vi "Find Resource by Type (U32).vi"(6 "Error if not found? (F)":bool, 8 "error in (no error)":errorcluster, 10 "Resource Type":u32, 11 "Resources":T2) -> (0 "error out":errorcluster, 1 "Index":i32, 2 "Found?":bool, 3 "Resource":T1)   [LabVIEW 2023]
uses:
  CTLs/Resource Array.ctl
  CTLs/Resource.ctl
  <vilib>/Utility/error.llb/Error Cluster From Error Code.vi
  <vilib>/ErrorRing/Error Ring.xnode
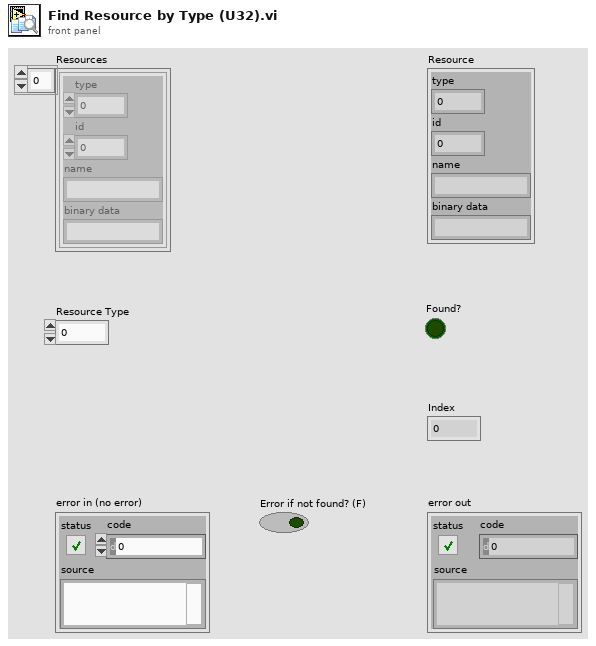
[diagram p1: front panel]
types:
  T1 = typedef "Resource.ctl" = cluster{"type":u32, "id":i32, "name":string, "binary data":string}
  T2 = typedef "Resource Array.ctl" = T1[]
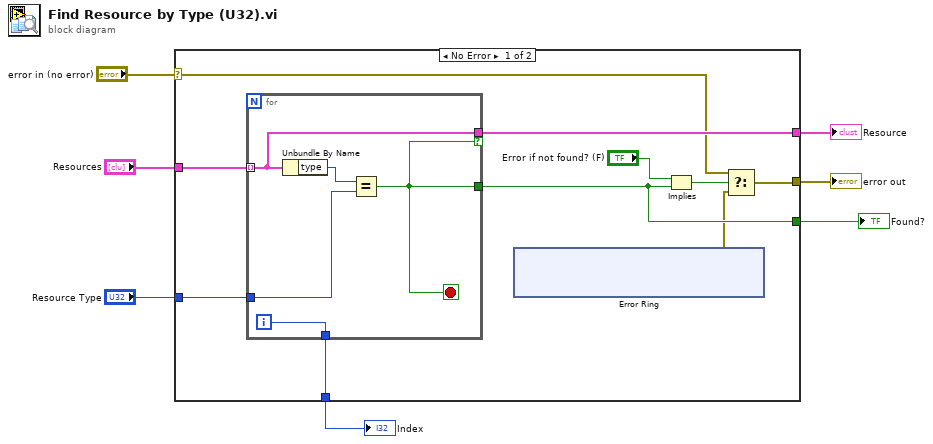
[diagram p0: block diagram]
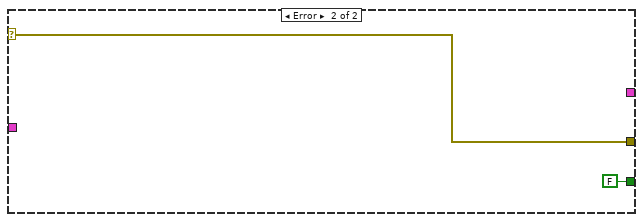
[diagram p2: hidden frame]
diagram:
  n1 = case shown="No Error" "error in (no error)" {
    selector: "error in (no error)" -> [w11 w28]
    tunnel: "Resources" -> [w17 _]
    tunnel: "Resource Type" -> [w16 _]
    tunnel: [w13 _] -> w5
    tunnel: [w12 _] -> w4
    tunnel: [w10 FALSE] -> w2
    tunnel: [w8 w28] -> w1
    frame No Error {
      n2 = for {
        tunnel: w17 -> [w24] mode=indexing
        tunnel: w16 -> [w25]
        tunnel: [w23] -> w10
        tunnel: [w24] -> w12 if=w23
        tunnel: [w22] -> w13
        i -> [w22]
        stop <- w23 stop-if-true
        n3 = Unbundle By Name(w24) -> ("type"=w26:u32)
        n4 = Equal?(x=w26, y=w25) -> (x = y?=w23:bool)
      }
      n5 = xnode "Error Ring"() -> ("error out"=w9:errorcluster)
      n6 = Implies(1:w10, 2:"Error if not found? (F)") -> (0:w14:bool)
      n7 = Select(t=w11, s=w14, f=w9) -> (s? t:f=w8:errorcluster)
    }
    frame Error {
    }
  }
  "error out" <- w1
  "Index" <- w5
  "Resource" <- w4
  "Found?" <- w2
